vi "Enqueue Change to Edge Cost.vi"(5 "cost":dbl=inf, 7 "error in (no error)":errorcluster, 8 "end node":string, 9 "start node":string, 10 "map reference in":refnum<data-value>) -> (0 "error out":errorcluster, 3 "map reference out":refnum<data-value>)   [LabVIEW 2017, in "NI_Robotics_DirectedGraphWorldMap.lvclass"]
doc: "Requests that LabVIEW set the <B>cost</B> of traversing the area of the directed graph map between <B>start node</B> and <B>end node</B> to the value you specify."
uses:
  <vilib>/robotics/Navigation/shared/WorldMap/DirectedGraphWorldMap/NI_Robotics_DirectedGraphWorldMap.lvclass
  <vilib>/robotics/Navigation/shared/WorldMap/DirectedGraphWorldMap/NI_Robotics_DirectedGraphWorldMap.lvclass/NI_Robotics_DirectedGraphWorldMap.ctl
  <vilib>/robotics/Utilities/NI_Robotics Utilities.lvlib
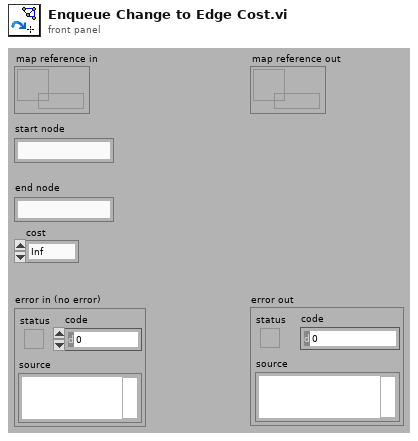
[diagram p1: front panel]
types:
  T1 = cluster{"start node":string, "end node":string, "cost":dbl}
  T2 = cluster{"Start":string, "End":string, "Cost":dbl}[]
  T3 = cluster{"start node":string, "end node":string, "cost":dbl}[]
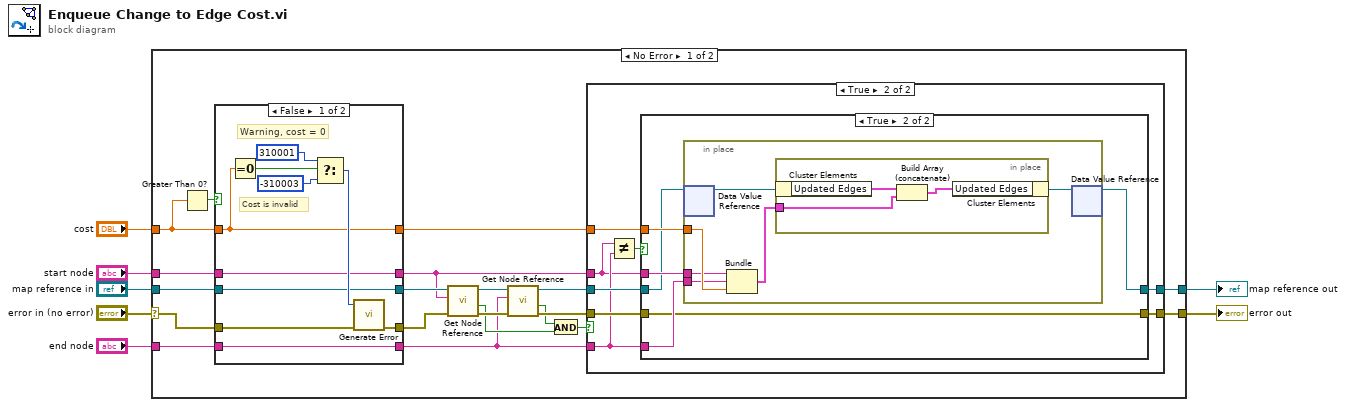
[diagram p0: block diagram]
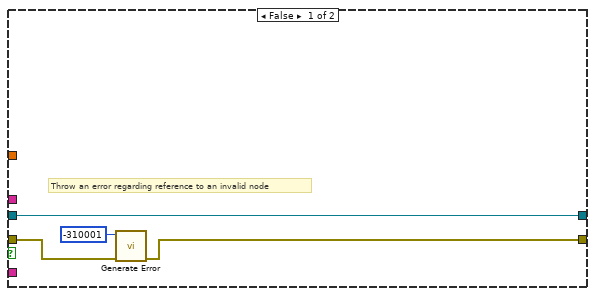
[diagram p3: hidden frame]
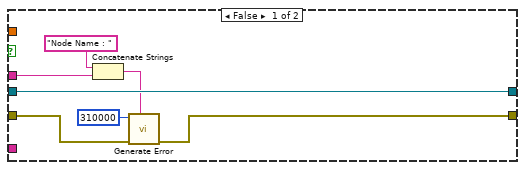
[diagram p4: hidden frame]
diagram:
  n1 = case shown="No Error" "error in (no error)" {
    selector: "error in (no error)" -> [w15 w78]
    tunnel: "start node" -> [w8 _]
    tunnel: "end node" -> [w12 _]
    tunnel: "cost" -> [w17 _]
    tunnel: [w22 w78] -> w4
    tunnel: "map reference in" -> [w10 w77]
    tunnel: [w19 w77] -> w2
    frame No Error {
      n2 = Greater Than 0?(x=w17) -> (x > 0?=w16:bool)
      n3 = case shown="False" w16 {
        tunnel: [w33 w42] -> w14
        tunnel: w15 -> [w34 w42]
        tunnel: [w31 w41] -> w18
        tunnel: w17 -> [w31 w41]
        tunnel: [w30 w40] -> w13
        tunnel: w12 -> [w30 w40]
        tunnel: [w29 w39] -> w11
        tunnel: w10 -> [w29 w39]
        tunnel: [w28 w38] -> w9
        tunnel: w8 -> [w28 w38]
        frame False {
          # "Warning, cost = 0"
          # "Cost is invalid"
          n4 = Equal To 0?(x=w31) -> (x = 0?=w37:bool)
          n5 = Select(t=310001 ("code"), s=w37, f=-310003 ("code")) -> (s? t:f=w32:i32)
          n6 = call <vilib>:"Generate Error.vi"("error in (no error)"=w34, "code"=w32) -> ("error out"=w33:errorcluster)  [unwired: 9 in]
        }
        frame True {
        }
      }
      n7 = call <vilib>:"Get Node Reference.vi"("error in (no error)"=w14, "name"=w9, "map reference in"=w11) -> ("error out"=w25:errorcluster, "found?"=w20:bool, "map reference out"=w27:refnum<data-value>)  [unwired: 5 in, 1 out]
      n8 = call <vilib>:"Get Node Reference.vi"("error in (no error)"=w25, "name"=w13, "map reference in"=w27) -> ("error out"=w24:errorcluster, "found?"=w21:bool, "map reference out"=w26:refnum<data-value>)  [unwired: 5 in, 1 out]
      n9 = And(x=w21, y=w20) -> (x .and. y?=w23:bool)
      n10 = case shown="True" w23 {
        tunnel: [w46 w52] -> w19
        tunnel: w26 -> [w46 w53]
        tunnel: w24 -> [w45 w51]
        tunnel: w18 -> [_ w54]
        tunnel: [w44 w50] -> w22
        tunnel: w9 -> [_ w47]
        tunnel: w13 -> [_ w48]
        frame False {
          # "Throw an error regarding reference to an invalid node"
          n11 = call <vilib>:"Generate Error.vi"("error in (no error)"=w45, "code"=-310001) -> ("error out"=w44:errorcluster)  [unwired: 9 in]
        }
        frame True {
          n12 = Not Equal?(x=w47, y=w48) -> (x != y?=w49:bool)
          n13 = case shown="True" w49 {
            tunnel: w54 -> [_ w67]
            tunnel: w47 -> [w56 w66]
            tunnel: w48 -> [_ w65]
            tunnel: w53 -> [w61 w64]
            tunnel: [w61 w63] -> w52
            tunnel: w51 -> [w60 w62]
            tunnel: [w59 w62] -> w50
            frame False {
              n14 = Concatenate Strings("Node Name : ", w56) -> (w55:string)
              n15 = call <vilib>:"Generate Error.vi"("<append> (\"\")"=w55, "error in (no error)"=w60, "code"=310000) -> ("error out"=w59:errorcluster)  [unwired: 8 in]
            }
            frame True {
              n16 = in-place {
                in-place-border: w67 -> [w73]
                in-place-border: w66 -> [w71]
                in-place-border: w65 -> [w70]
                n17 = in-place-dvr #1(w64) -> (w68:refnum<class "NI_Robotics_DirectedGraphWorldMap.lvclass">)  [unwired: 1 out]
                n18 = Bundle("start node"=w71, "end node"=w70, "cost"=w73) -> (w72:T1)  [unwired: 1 in]
                n19 = in-place {
                  in-place-border: w72 -> [w74]
                  n20 = in-place-cluster #2(w68) -> ("Updated Edges"=w76:T2)
                  n21 = Build Array (concatenate)(w76, w74) -> (w75:T3)
                  n22 = in-place-cluster #2("Updated Edges"=w75) -> (w69:refnum<class "NI_Robotics_DirectedGraphWorldMap.lvclass">)
                }
                n23 = in-place-dvr #1(w69) -> (w63:refnum<data-value>)  [unwired: 1 out]
              }
            }
          }
        }
      }
    }
    frame Error {
    }
  }
  "map reference out" <- w2
  "error out" <- w4
